vi "Log Start Inspect State.vi"(4 "Speed":u16, 6 "Start Collect (Reply Payload)":T2, 7 "Data Collect Params":T1, 8 "error in (no error)":errorcluster, 9 "Timed out?":bool, 10 "Laser On":bool, 11 "EventLog in":refnum<class "EventLog.lvclass">) -> (0 "error out":errorcluster, 3 "EventLog out":refnum<class "EventLog.lvclass">)   [LabVIEW 2015, in "Tool Module.lvlib"]
uses:
  Tool Module.lvlib
  Collect Data Mgr/Start Collect (Reply Payload)--cluster.ctl
  Collect Data Mgr/Data Collect Parameters typedef--cluster.ctl
  Event Logger Library/Event Log/EventLog.lvclass
  Collect Data Mgr/Collect Data Mgr.lvlib
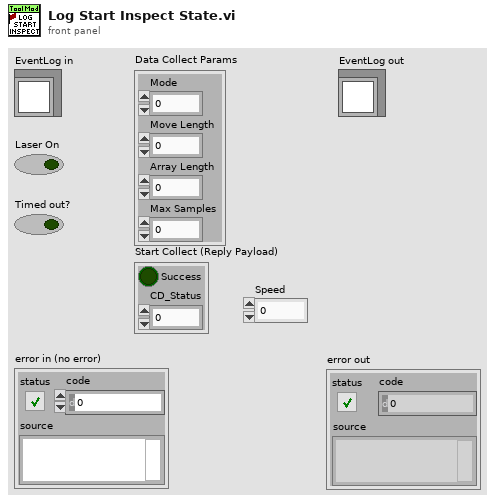
[diagram p1: front panel]
types:
  T1 = typedef "Collect Data Mgr.lvlib/Data Collect Parameters typedef--cluster.ctl" = cluster{"Mode":i8, "Move Length":i32, "Array Length":i32, "Max Samples":i32}
  T2 = typedef "Collect Data Mgr.lvlib/Start Collect (Reply Payload)--cluster.ctl" = cluster{"Success":bool, "CD_Status":u8}
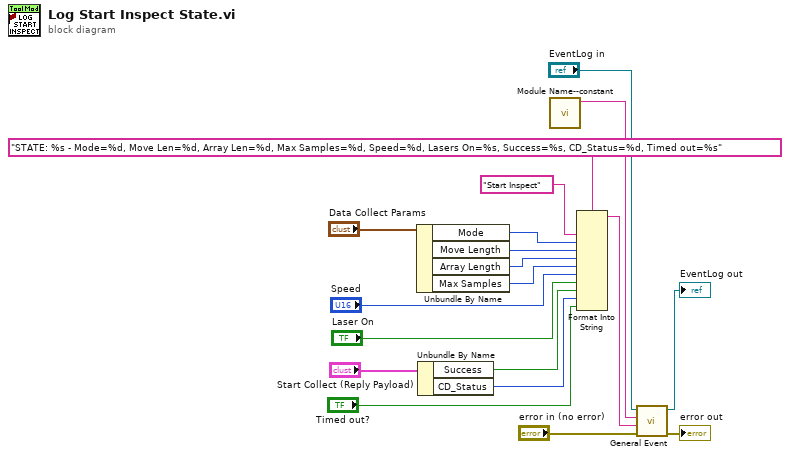
[diagram p0: block diagram]
diagram:
  n1 = Unbundle By Name("Data Collect Params") -> ("Mode"=w10:i8, "Move Length"=w11:i32, "Array Length"=w12:i32, "Max Samples"=w13:i32)
  n2 = Unbundle By Name("Start Collect (Reply Payload)") -> ("Success"=w17:bool, "CD_Status"=w18:u8)
  n3 = call "Module Name--constant.vi"() -> ("Module Name"=w2:string)  [unwired: 11 in]
  n4 = Format Into String(format string="STATE: %s - Mode=%d, Move Len=%d, Array Len=%d, Max Samples=%d, Speed=%d, Lasers On=%s, Success=%s, CD_Status=%d, Timed out=%s", "Start Inspect", w10, w11, w12, w13, "Speed", "Laser On", w17, w18, "Timed out?") -> (resulting string=w8:string)  [unwired: 2 in, 1 out]
  n5 = call "General Event.vi"("error in (no error)"="error in (no error)", "Event Description"=w8, "Event Name"=w2, "EventLog ref"="EventLog in") -> ("error out"=→"error out":errorcluster, "EventLog ref"=→"EventLog out":refnum<class "EventLog.lvclass">)  [unwired: 6 in]
